vi "LCR_Readout.vi"(8 "error in (no error)":errorcluster, 10 "Frequency in Hz":i32, 11 "WK6440B in":refnum<class "WK6440B.lvclass">) -> (0 "error out":errorcluster, 1 "Resistance in Ohm":dbl, 2 "Capacitance in pF":dbl, 3 "WK6440B out":refnum<class "WK6440B.lvclass">)   [LabVIEW 2019, in "WK6440B.lvclass"]
uses:
  WK6440B.lvclass
  C:/Users/Semiprobe/Desktop/Probe-Test-Software/itk-strip-sensor-qc/LabVIEW 2019/InstrControl/InstrControl.lvclass
  QCtests/general_VIs/globals/QC_RunInformation.vi
  InstrControl.lvclass
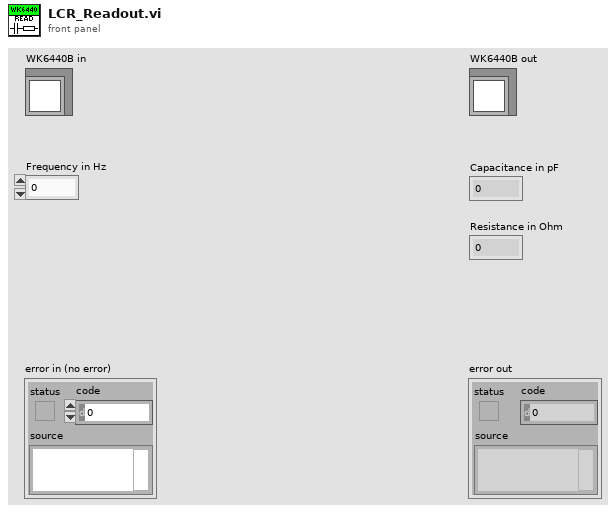
[diagram p1: front panel]
types:
  T1 = cluster{"Sensor Serial No.:":string, "Wafer Serial No.:":string, "Batch:":string, "Manufacturer:":string, "Device Category:":string, "Database Serial No.:":string, "Date Initiated:":string, "Time Initiated:":string, "Test":string, "Instruments used:":string, "Probeplan used:":string, "End of Run comment:":string, "User:":string}
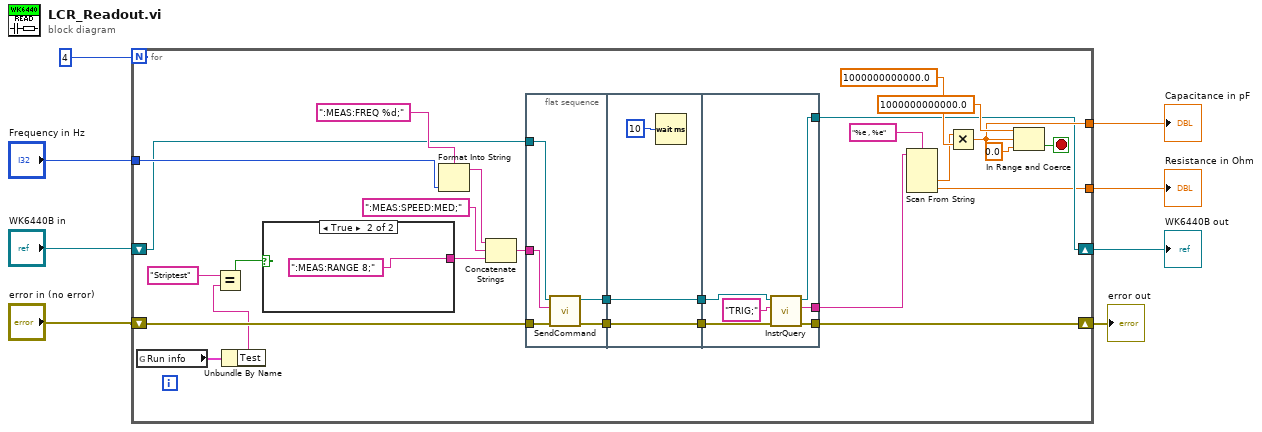
[diagram p0: block diagram]
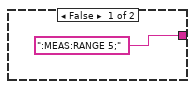
[diagram p2: hidden frame]
diagram:
  n1 = for {
    N: 4 -> [_]
    tunnel: [w14] -> w4
    tunnel: [w32] -> w5
    tunnel: "Frequency in Hz" -> [w30]
    shift-right: [w15] -> w1
    shift-left: "WK6440B in" -> [w22]
    shift-right: [w20] -> w6
    shift-left: "error in (no error)" -> [w29]
    stop <- w31 stop-if-true
    n2 = global read "QC_RunInformation.vi" "Run info"() -> (w13:T1)
    n3 = Unbundle By Name(w13) -> ("Test"=w12:string)
    n4 = Equal?(x="Striptest", y=w12) -> (x = y?=w10:bool)
    n5 = case shown="True" w10 {
      tunnel: [":MEAS:RANGE 5;" ":MEAS:RANGE 8;"] -> w9
      frame False {
      }
      frame True {
      }
    }
    n6 = Format Into String(format string=":MEAS:FREQ %d;", w30) -> (resulting string=w28:string)  [unwired: 2 in, 1 out]
    n7 = Concatenate Strings(w28, ":MEAS:SPEED:MED;", w9) -> (w35:string)
    n8 = flat-sequence {
      tunnel: w35 -> [w40]
      tunnel: w29 -> [w42]
      tunnel: w22 -> [w38]
      tunnel: [w41] -> w19
      tunnel: [w39] -> w17
      tunnel: w19 -> [w44]
      tunnel: [w44] -> w18
      tunnel: w17 -> [w43]
      tunnel: [w43] -> w16
      tunnel: [w50] -> w20
      tunnel: [w49] -> w21
      tunnel: w18 -> [w51]
      tunnel: w16 -> [w47]
      tunnel: [w46] -> w15
      frame #0 {
        n9 = call "SendCommand.vi"("error in (no error)"=w42, "Command string"=w40, "InstControl in"=w38) -> ("error out"=w41:errorcluster, "InstControl out"=w39:refnum<class "WK6440B.lvclass">)  [unwired: 7 in]
      }
      frame #1 {
        n10 = Wait (ms)(milliseconds to wait=10) -> ()  [unwired: 1 out]
      }
      frame #2 {
        n11 = call-dynamic "InstrQuery.vi"("error in (no error)"=w51, "Command string"="TRIG;", "InstControl in"=w47) -> ("error out"=w50:errorcluster, "Instrument response"=w49:string, "InstControl out"=w46:refnum<class "WK6440B.lvclass">)  [unwired: 6 in]
      }
    }
    n12 = Scan From String(format string="%e , %e", input string=w21) -> (output 1=w23:dbl, output 2=w14:dbl)  [unwired: 4 in, 3 out]
    n13 = Multiply(x=w23, y=1000000000000.0) -> (x*y=w32:dbl)
    n14 = In Range and Coerce(upper limit=1000000000000.0 ("y"), x=w32, lower limit=0.0) -> (In Range?=w31:bool)  [unwired: 1 out]
  }
  "error out" <- w6
  "WK6440B out" <- w1
  "Capacitance in pF" <- w5
  "Resistance in Ohm" <- w4
